vi "Read Channel Single Shot (Volts).vi"(8 "error in (no error)":errorcluster, 10 "ADC Channel Selection":T1, 11 "LINX-ADS1256 in":refnum<class "LINX-ADS1256.lvclass">) -> (0 "error out":errorcluster, 2 "ADC Volts":dbl, 3 "LINX-ADS1256 out":refnum<class "LINX-ADS1256.lvclass">)   [LabVIEW 2020, in "LINX-ADS1256.lvclass"]
uses:
  LINX-ADS1256.lvclass
  Channel Selection.ctl
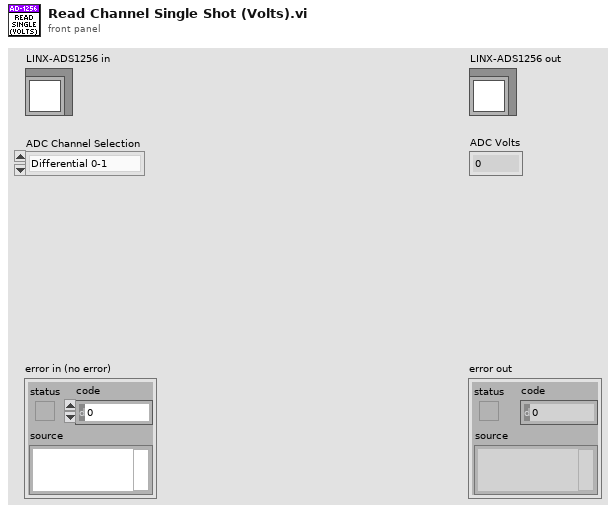
[diagram p1: front panel]
types:
  T1 = typedef "LINX-ADS1256.lvclass/Channel Selection.ctl" = enum16{"Differential 0-1", "Differential 2-3", "Differential 4-5", "Differential 6-7", "Single Ended 0", "Single Ended 1", "Single Ended 2", "Single Ended 3", "Single Ended 4", "Single Ended 5", "Single Ended 6", "Single Ended 7"}
  T2 = typedef "LINX-ADS1256.lvclass/Programmable Gain Selection.ctl" = enum16{"+/-5V (1)", "+/-2.5V (2)", "+/-1.25V (4)", "+/-0.625V (8)", "+/-312.5mV (16)", "+/-156.25mV (32)", "+/-78.125mV (64)"}
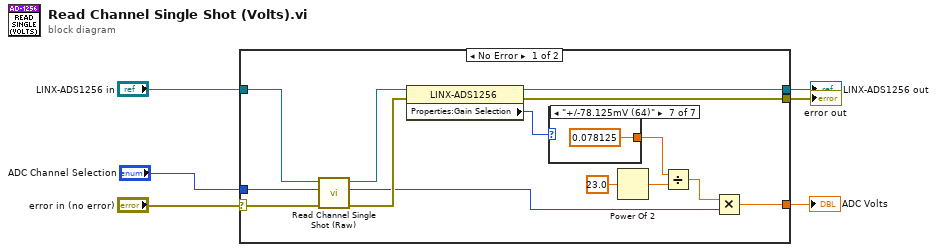
[diagram p0: block diagram]
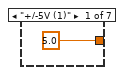
[diagram p2: hidden frame]
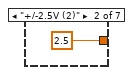
[diagram p3: hidden frame]
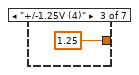
[diagram p4: hidden frame]
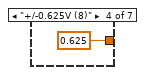
[diagram p5: hidden frame]
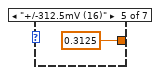
[diagram p6: hidden frame]
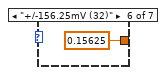
[diagram p7: hidden frame]
diagram:
  n1 = case shown="No Error" "error in (no error)" {
    selector: "error in (no error)" -> [w20 w29]
    tunnel: [w10 w29] -> w5
    tunnel: [w15 w28] -> w3
    tunnel: "LINX-ADS1256 in" -> [w19 w28]
    tunnel: "ADC Channel Selection" -> [w18 _]
    tunnel: [w9 _] -> w1
    frame No Error {
      n2 = call "Read Channel Single Shot (Raw).vi"("error in (no error)"=w20, "ADC Channel Selection"=w18, "LINX-ADS1256 in"=w19) -> ("error out"=w16:errorcluster, "ADC Raw"=w11:i32, "LINX-ADS1256 out"=w17:refnum<class "LINX-ADS1256.lvclass">)  [unwired: 6 in]
      n3 = property class="LINX-ADS1256"(reference=w17, error in=w16) -> (reference out=w15:refnum<class "LINX-ADS1256.lvclass">, error out=w10:errorcluster, "Properties:Gain Selection"=w8:T2)
      n4 = case shown="\"+/-78.125mV (64)\"" w8 {
        tunnel: [5.0 2.5 1.25 0.625 0.3125 0.15625 0.078125] -> w7
        frame "+/-5V (1)" {
        }
        frame "+/-2.5V (2)" {
        }
        frame "+/-1.25V (4)" {
        }
        frame "+/-0.625V (8)" {
        }
        frame "+/-312.5mV (16)" {
        }
        frame "+/-156.25mV (32)" {
        }
        frame "+/-78.125mV (64)" {
        }
      }
      n5 = Power Of 2(x=23.0) -> (2^x=w14:dbl)
      n6 = Divide(x=w7, y=w14) -> (x/y=w13:dbl)
      n7 = Multiply(x=w13, y=w11) -> (x*y=w9:dbl)
    }
    frame Error {
    }
  }
  "error out" <- w5
  "LINX-ADS1256 out" <- w3
  "ADC Volts" <- w1
